vi "Config ARB IQ Modulation.vi"(0 "VISA Resource Name":refnum<visa-resource-name>, 1 "Filter Auto (T: ON)":bool=TRUE, 2 "Filter (2: THROUGH)":enum16{"2.1 MHz", "40.0 MHz", "THROUGH"}(ring)=enum."THROUGH", 5 "Standard (0: IS-95A)":T1(ring), 7 "Attenuation Auto (T: ON)":bool=TRUE, 9 "Attenuation (2.0)":dbl=2.0, 11 "error in (no error)":errorcluster {"code" format="%.0x"}, 12 "External Filter Auto (T: ON)":bool=TRUE, 13 "External Filter (1: THROUGH)":enum16{"40.0 MHz", "THROUGH"}(ring)=enum."THROUGH") -> (4 "VISA Resource Name Out":refnum<visa-resource-name>, 15 "error out":errorcluster {"code" format="%.0x"})   [LabVIEW 2012, in "Agilent ESG Series.lvlib"]
doc: "This VI configures the I/Q modulation signals for CDMA arbitrary system.\n\nNotes:\n(1) This VI is valid only on instrument E4438C."
uses:
  <instrlib>/Agilent ESG Series/Agilent ESG Series.lvlib
panel:
  # "ON"
  # "OFF"
  # "ON"
  # "OFF"
  # "ON"
  # "OFF"
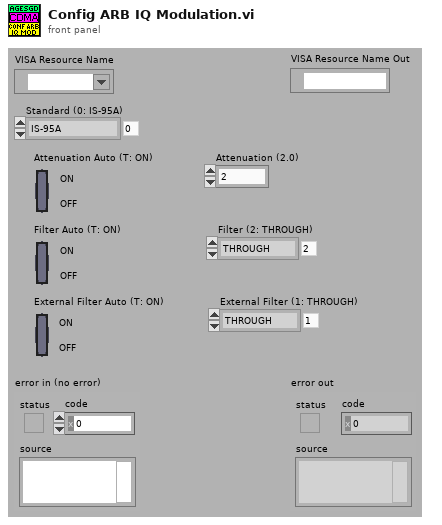
[diagram p1: front panel]
types:
  T1 = enum16{"IS-95A", "CDMA2000", "WCDMA", "Dual Arbitrary"}
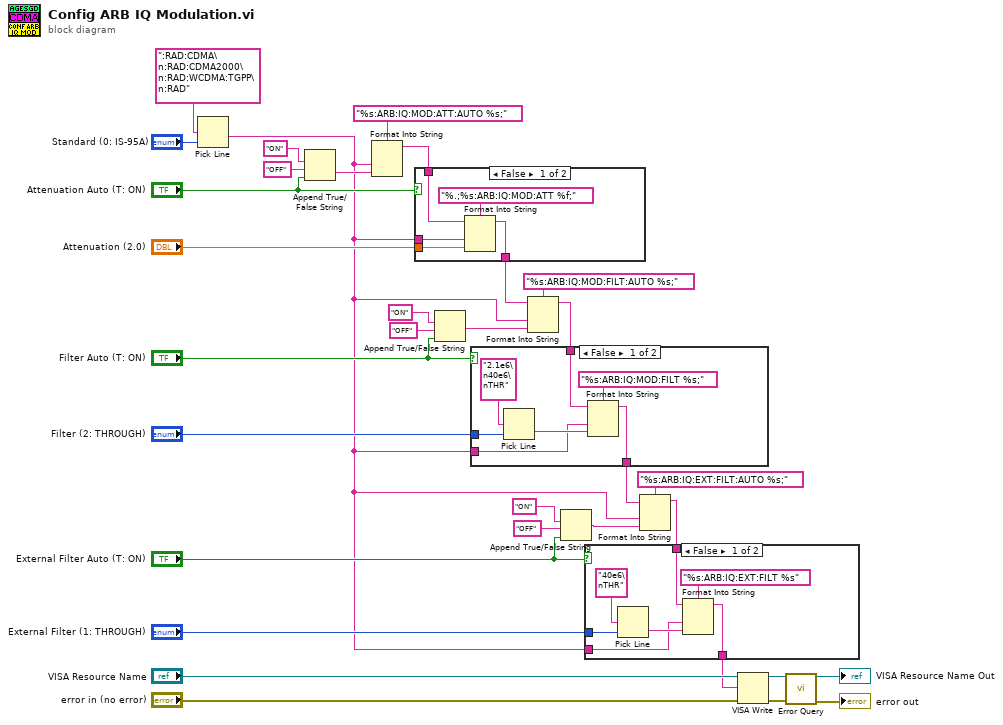
[diagram p0: block diagram]
diagram:
  n1 = Pick Line(multi-line string=":RAD:CDMA\n:RAD:CDMA2000\n:RAD:WCDMA:TGPP\n:RAD", line index="Standard (0: IS-95A)") -> (output string=w1:string)  [unwired: 1 in]
  n2 = Append True/False String(1:"Attenuation Auto (T: ON)", 2:"OFF" ("false string"), 3:"ON" ("multi-line string")) -> (0:w4:string)  [unwired: 1 in]
  n3 = Format Into String(format string="%s:ARB:IQ:MOD:ATT:AUTO %s;", w1, w4) -> (resulting string=w13:string)  [unwired: 2 in, 1 out]
  n4 = case shown="False" "Attenuation Auto (T: ON)" {
    tunnel: "Attenuation (2.0)" -> [w35 _]
    tunnel: w13 -> [w37 w39]
    tunnel: [w36 w39] -> w12
    tunnel: w1 -> [w34 _]
    frame False {
      n5 = Format Into String(format string="%.;%s:ARB:IQ:MOD:ATT %f;", initial string=w37, w34, w35) -> (resulting string=w36:string)  [unwired: 1 in, 1 out]
    }
    frame True {
    }
  }
  n6 = Append True/False String(1:"Filter Auto (T: ON)", 2:"OFF" ("false string"), 3:"ON" ("multi-line string")) -> (0:w2:string)  [unwired: 1 in]
  n7 = Format Into String(format string="%s:ARB:IQ:MOD:FILT:AUTO %s;", initial string=w12, w1, w2) -> (resulting string=w11:string)  [unwired: 1 in, 1 out]
  n8 = case shown="False" "Filter Auto (T: ON)" {
    tunnel: "Filter (2: THROUGH)" -> [w45 _]
    tunnel: w11 -> [w43 w47]
    tunnel: [w42 w47] -> w10
    tunnel: w1 -> [w40 _]
    frame False {
      n9 = Pick Line(multi-line string="2.1e6\n40e6\nTHR", line index=w45) -> (output string=w41:string)  [unwired: 1 in]
      n10 = Format Into String(format string="%s:ARB:IQ:MOD:FILT %s;", initial string=w43, w40, w41) -> (resulting string=w42:string)  [unwired: 1 in, 1 out]
    }
    frame True {
    }
  }
  n11 = Append True/False String(1:"External Filter Auto (T: ON)", 2:"OFF" ("false string"), 3:"ON" ("multi-line string")) -> (0:w3:string)  [unwired: 1 in]
  n12 = Format Into String(format string="%s:ARB:IQ:EXT:FILT:AUTO %s;", initial string=w10, w1, w3) -> (resulting string=w9:string)  [unwired: 1 in, 1 out]
  n13 = case shown="False" "External Filter Auto (T: ON)" {
    tunnel: "External Filter (1: THROUGH)" -> [w54 _]
    tunnel: w9 -> [w51 w55]
    tunnel: [w50 w55] -> w8
    tunnel: w1 -> [w48 _]
    frame False {
      n14 = Pick Line(multi-line string="40e6\nTHR", line index=w54) -> (output string=w49:string)  [unwired: 1 in]
      n15 = Format Into String(format string="%s:ARB:IQ:EXT:FILT %s", initial string=w51, w48, w49) -> (resulting string=w50:string)  [unwired: 1 in, 1 out]
    }
    frame True {
    }
  }
  n16 = VISA Write(VISA resource name="VISA Resource Name", write buffer=w8, error in (no error)="error in (no error)") -> (VISA resource name out=w29:refnum<visa-resource-name>, error out=w28:errorcluster)  [unwired: 1 out]
  n17 = call <instrlib>:"Error Query.vi"("VISA Resource Name"=w29, "error in (no error)"=w28) -> ("VISA Resource Name Out"=→"VISA Resource Name Out":refnum<visa-resource-name>, "error out"=→"error out":errorcluster)  [unwired: 10 in, 2 out]
